vi "incrementCalc.vi"(8 "End":dbl, 9 "Start":dbl, 10 "#Steps":i32) -> (1 "Invalid?":bool, 2 "Increment":dbl)   [LabVIEW 2015]
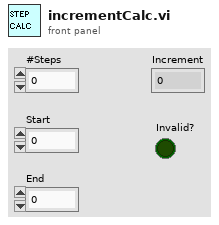
[diagram p1: front panel]
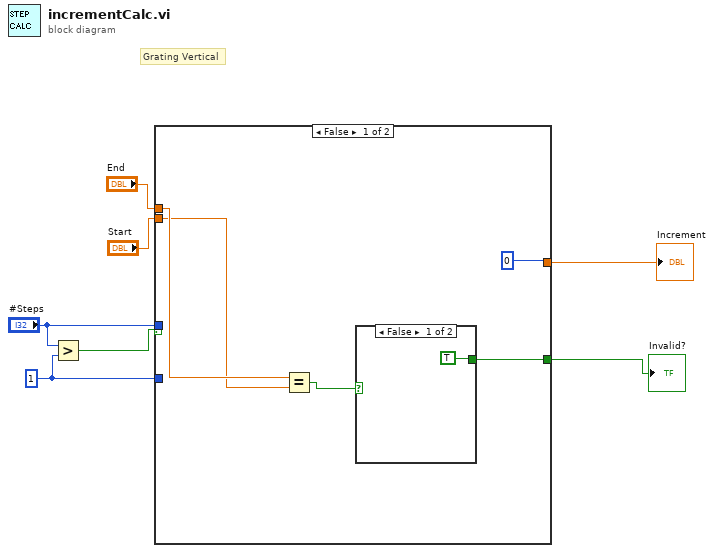
[diagram p0: block diagram]
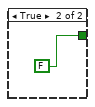
[diagram p2: hidden frame]
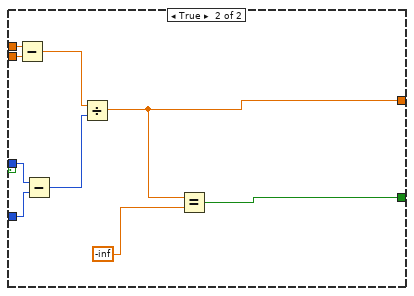
[diagram p3: hidden frame]
diagram:
  w5 = 1
  # "Grating Vertical"
  n1 = Greater?(x="#Steps", y=w5) -> (0:w3:bool)
  n2 = case shown="False" w3 {
    tunnel: "End" -> [w10 w23]
    tunnel: "Start" -> [w9 w22]
    tunnel: w5 -> [_ w21]
    tunnel: "#Steps" -> [_ w20]
    tunnel: [0 w16] -> w2
    tunnel: [w8 w15] -> w1
    frame False {
      n3 = Equal?(x=w10, y=w9) -> (x = y?=w11:bool)
      n4 = case shown="False" w11 {
        tunnel: [TRUE FALSE] -> w8
        frame False {
        }
        frame True {
        }
      }
    }
    frame True {
      n5 = Subtract(x=w23, y=w22) -> (x-y=w18:dbl)
      n6 = Subtract(x=w20, y=w21) -> (x-y=w19:i32)
      n7 = Divide(x=w18, y=w19) -> (x/y=w16:dbl)
      n8 = Equal?(x=w16, y=-inf) -> (x = y?=w15:bool)
    }
  }
  "Increment" <- w2
  "Invalid?" <- w1
